vi "portClose.vi"(2 "error in (no error)":errorcluster, 3 "COMport":string="COM6") -> (0 "error out":errorcluster)   [LabVIEW 2015]
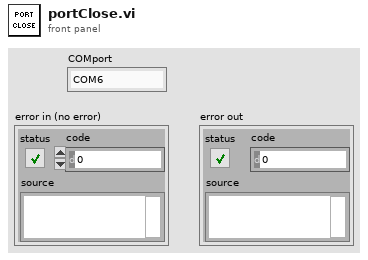
[diagram p1: front panel]
types:
  T1 = cluster{"OpenPort":bool, "ClosePort":bool, "Baudrate":i32, "Wait":u16, "ReadWrite":bool}
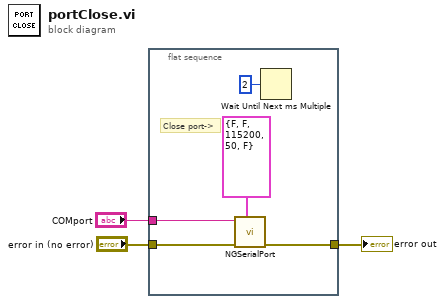
[diagram p0: block diagram]
diagram:
  n1 = flat-sequence {
    tunnel: [w7] -> w3
    tunnel: "error in (no error)" -> [w6]
    tunnel: "COMport" -> [w4]
    frame #0 {
      # "Close port->"
      n2 = call "NGSerialPort.vi"("PortParameters"=T1 {"OpenPort"=FALSE, "ClosePort"=FALSE, "Baudrate"=115200, "Wait"=50, "ReadWrite"=FALSE}, "error in"=w6, "VISA in"=w4) -> ("error out"=w7:errorcluster)  [unwired: 6 in, 2 out]
      n3 = Wait Until Next ms Multiple(millisecond multiple=u32 2) -> ()  [unwired: 1 out]
    }
  }
  "error out" <- w3
